vi "Protokoll.vi"() -> ()   [LabVIEW 2015, in "EPA 1065.lvlib" / "Interference verificaton 1065-366.lvlib"]
uses:
  Interference verificaton 1065-366.lvlib
  Allgemein/allgemeine Sub-VIs.lvlib
  Aktion FGV Test.ctl
  Aktion FGV Protokoll.ctl
  <vilib>/Waveform/WDTFileIO.llb/Read Waveform from File.vi
  Visualisierungs Elemente/String - Ausgabefeld.ctl
  Visualisierungs Elemente/Zahlen-Ausgabefeld.ctl
  Visualisierungs Elemente/Button.ctl
panel:
  out "Graph2 2":waveform(dbl)[](graph) caption="Graph2"
  out "Flow-weighted mean":T1
  out "Measured Concentration 3":T1
  out "Measured Concentration 2":T1
  out "Komponente 4":T1 caption="Interferent 3"
  out "Komponente 3":T1 caption="Interferent 2"
  out "Komponente 2":T1 caption="Interferent 1"
  out "Measured Interference %":T1
  in  "Screenshot":T2
  in  "OK":T2
  out "Allowed Interference":T1
  out "Measured Interference":T1
  out "Measured Concentration 1":T1
  out "Target Concentration 3":T1
  out "Target Concentration 2":T1
  out "Target Concentration 1":T1
  out "Datum / Uhrzeit":T1 caption="Date/Time"
  out "Boolesch":bool
  out "Ist Interference":T3 format="%#_5g"
  out "Soll Interference":T3 format="%#_5g"
  out "Konzentration berechnet":T3 caption="Concentration Calculated" format="%#_5g"
  out "Wasserkonzentration":T3 caption="Water-Concentration" format="%#_5g"
  out "Konzentration Feucht":T3 format="%#_5g"
  out "Konzentration Trocken":T3 format="%#_5g"
  out "Komponente":T1 caption="Component"
  out "Bearbeiter":T1 caption="Analyst"
  out "Graph2":waveform(dbl)[](graph)
  # "Interference Test"
  # "Interference Test"
  # "EPA §1065.366\n\nInterference verification of CH4, C2H6,"
  # "Evaluation"
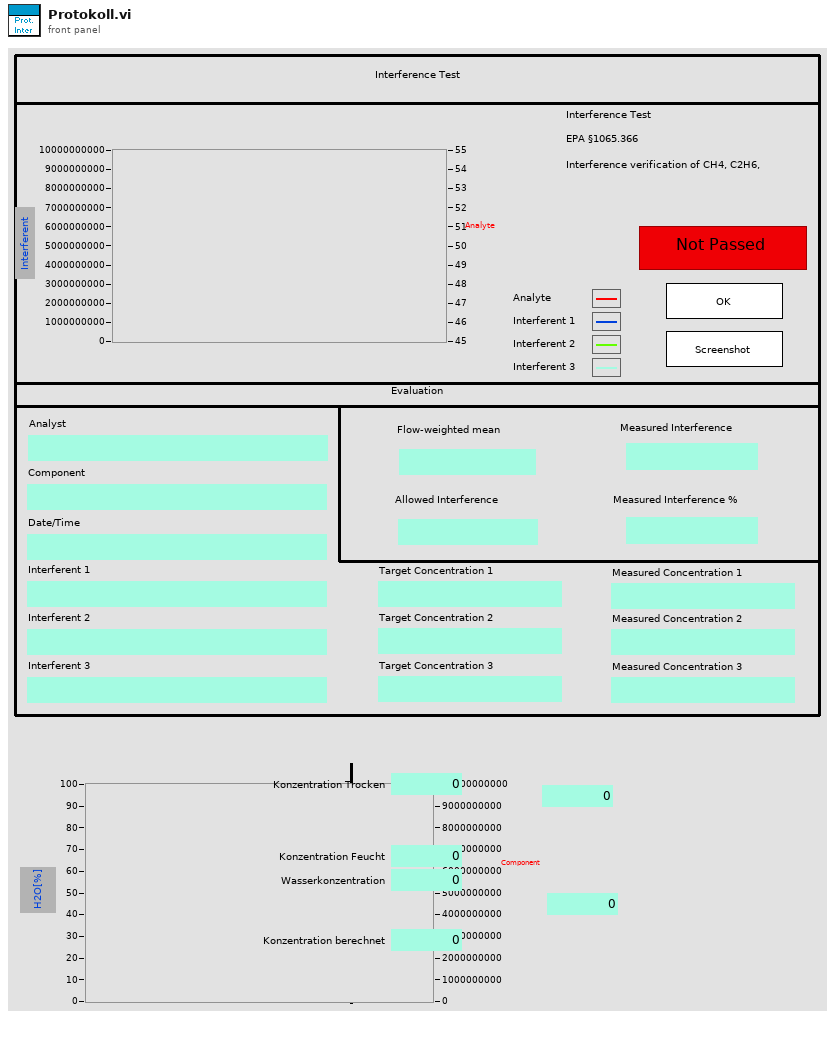
[diagram p1: front panel]
types:
  T1 = typedef "String - Ausgabefeld.ctl" = string
  T2 = typedef "Button.ctl" = bool
  T3 = typedef "Zahlen-Ausgabefeld.ctl" = sgl
  T4 = typedef "EPA 1065.lvlib/Interference verificaton 1065-366.lvlib/Aktion FGV Protokoll.ctl" = enum16{"Lesen", "ini"}
  T5 = typedef "EPA 1065.lvlib/Interference verificaton 1065-366.lvlib/Aktion FGV Test.ctl" = enum16{"Lesen", "ini", "Wasserkonzentration", "Wet", "Dry", "Ergebnis", "Graph", "Interference Daten", "Speichern"}
  T6 = typedef "imagedata.ctl" = cluster{"image type":i32, "image depth":i32, "image":u8[], "mask":u8[], "colors":u32[], "Rectangle":cluster{"left":i16, "top":i16, "right":i16, "bottom":i16}}
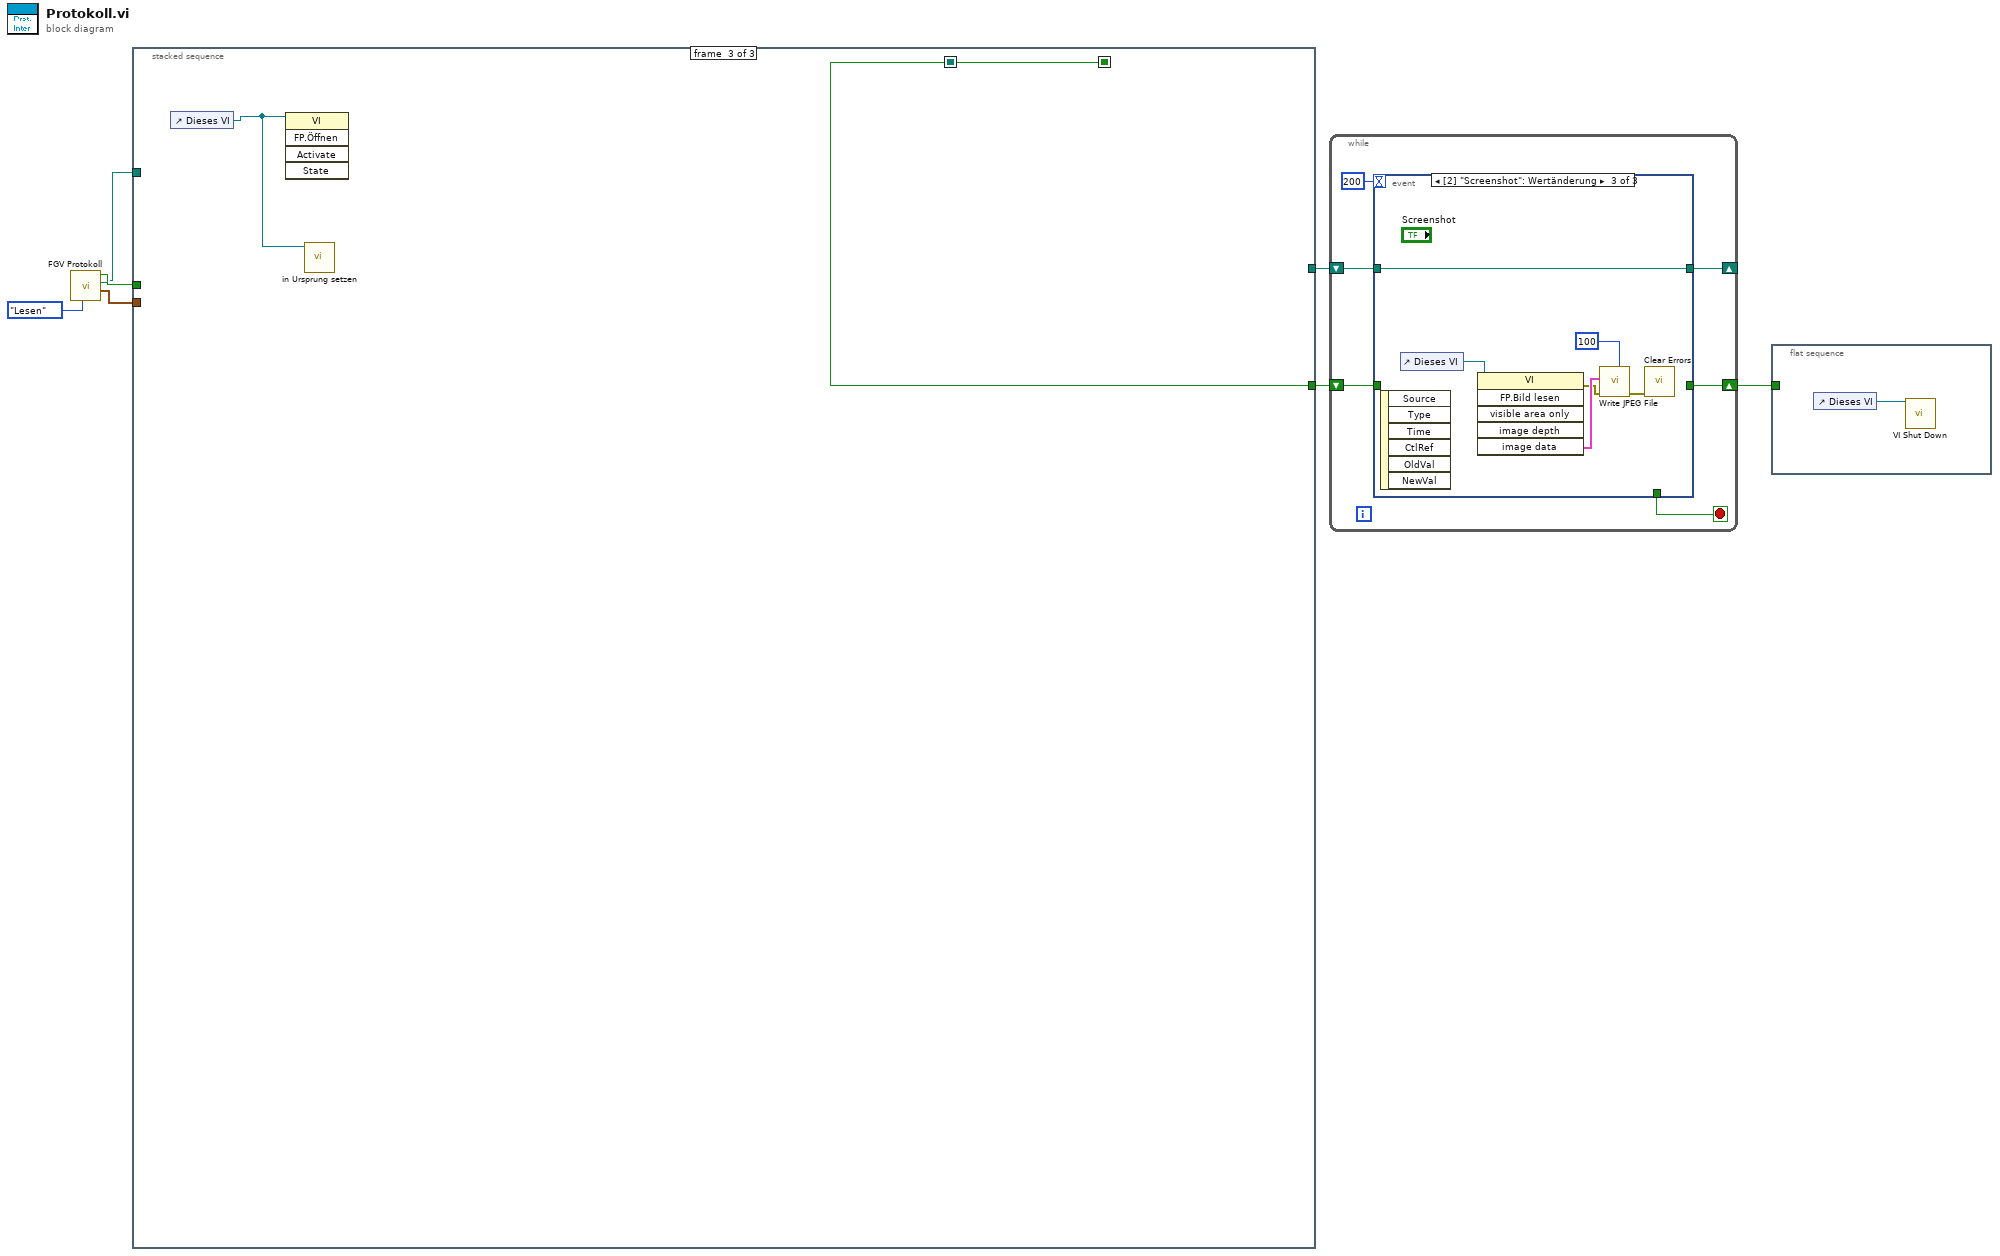
[diagram p0: block diagram]
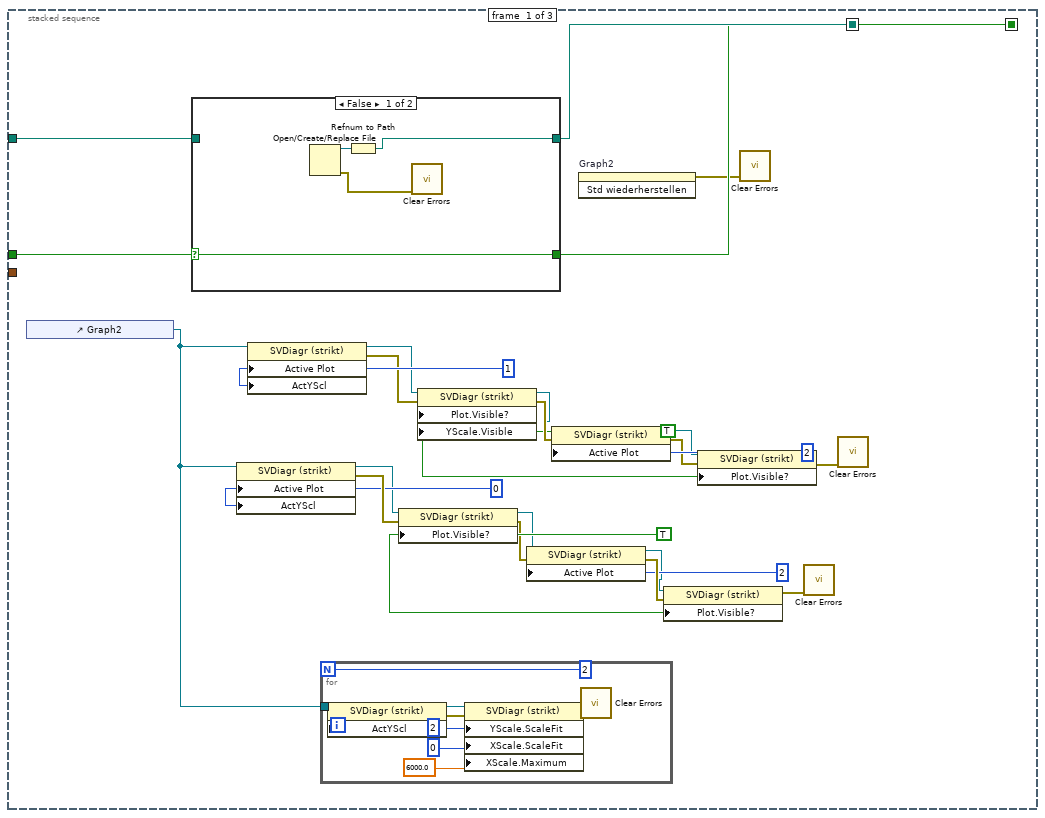
[diagram p2: hidden frame]
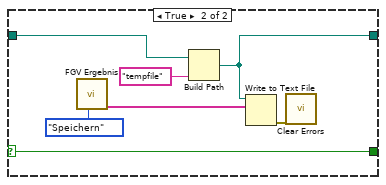
[diagram p3: hidden frame]
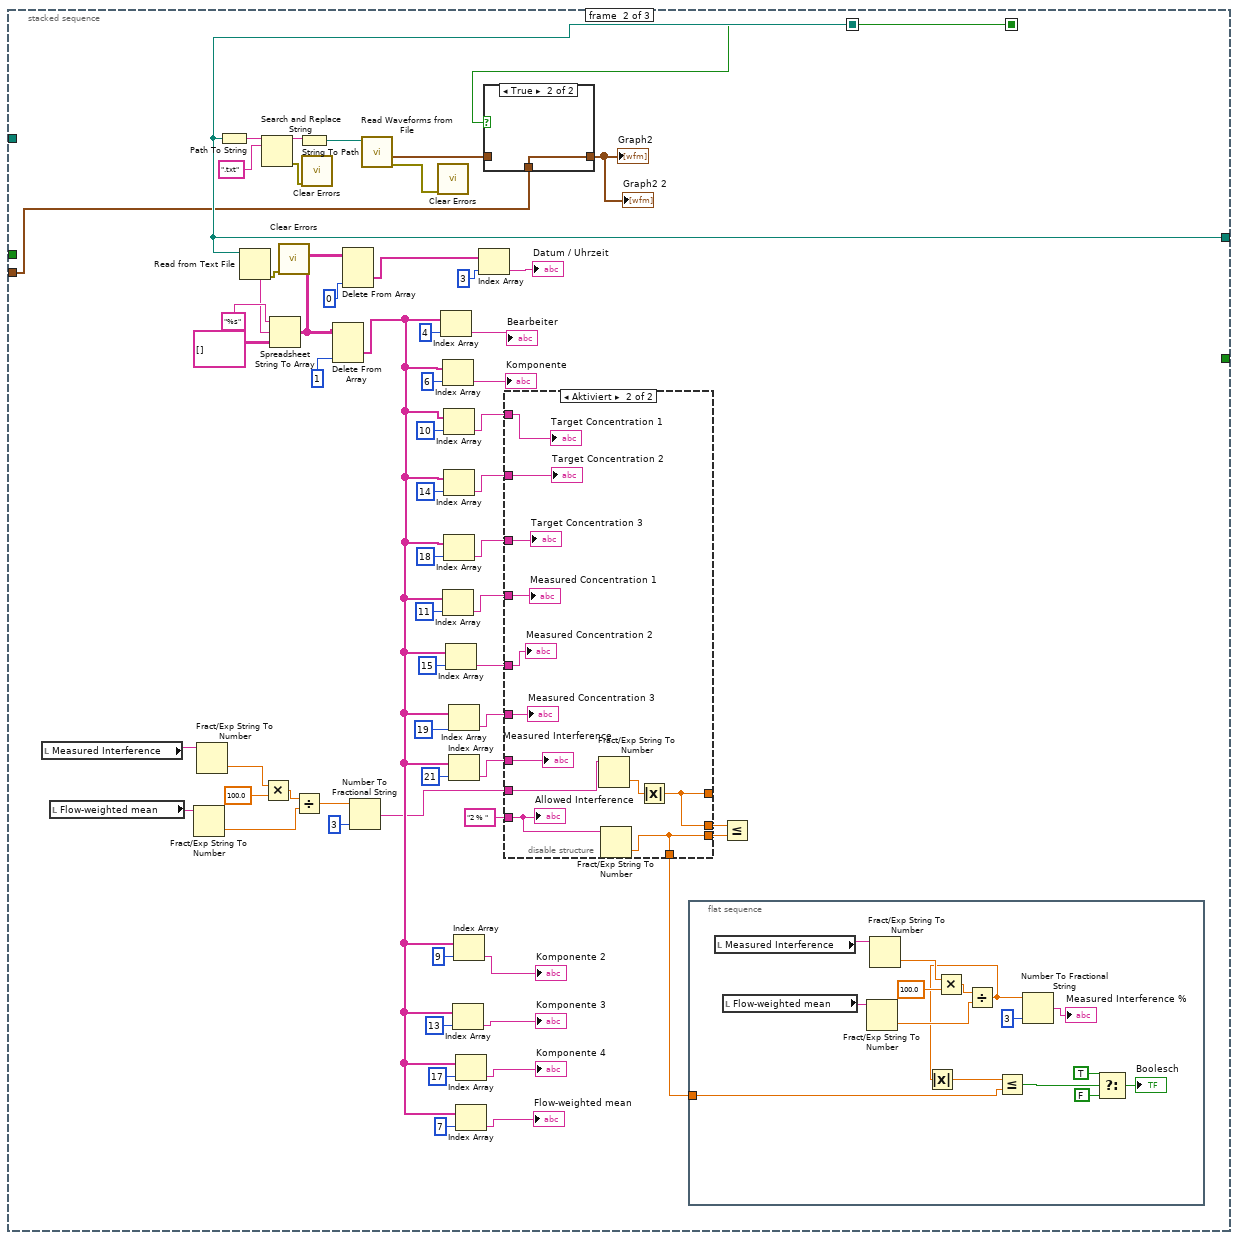
[diagram p4: hidden frame]
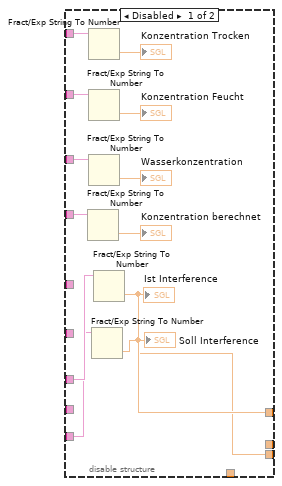
[diagram p6: hidden frame]
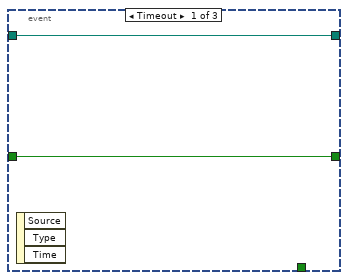
[diagram p7: hidden frame]
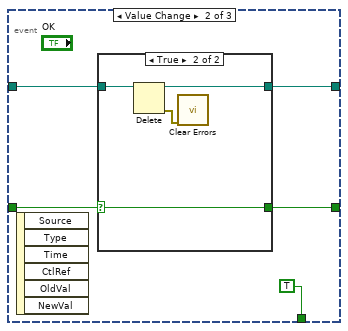
[diagram p8: hidden frame]
diagram:
  n1 = call "FGV Protokoll.vi"("Enum"=Aktion_FGV_Protokoll."Lesen") -> ("Graph2 2"=w1:waveform(dbl)[], "Pfad"=w2:path, "Boolesch 2"=w3:bool)  [unwired: 7 in, 1 out]
  n2 = stacked-sequence {
    seq-local: [w34 _ _] -> [_ w86 _]
    seq-local: [w33 _ _] -> [_ w82 w156]
    tunnel: [_ _ w156] -> w6
    tunnel: [_ w86 _] -> w5
    tunnel: w3 -> [w9 _ _]
    tunnel: w2 -> [w8 _ _]
    tunnel: w1 -> [_ w80 _]
    frame #0 {
      w25 = TRUE ("Plot.Sichtbar")
      w20 = u32 0 ("Aktiver Plot")
      w19 = TRUE ("Plot.Sichtbar")
      w32 = u32 1 ("Aktiver Plot")
      n3 = control-ref of="Graph2"() -> (w18:refnum<vi>)
      n4 = case shown="False" w9 {
        selector: w9 -> [w46 w51]
        tunnel: [w43 w48] -> w34
        tunnel: [w46 w51] -> w33
        tunnel: w8 -> [_ w47]
        frame False {
          n5 = Open/Create/Replace File() -> (refnum out=w45:refnum<file>, error out=w44:errorcluster)  [unwired: 6 in, 1 out]
          n6 = Refnum to Path(1:w45) -> (0:w43:path)
          n7 = call <vilib>:"Clear Errors.vi"("error in (no error)"=w44) -> ()  [unwired: 5 in, 2 out]
        }
        frame True {
          n8 = call "FGV Ergebnis.vi"("Enum"=Aktion_FGV_Test."Speichern") -> ("Protokoll"=w53:T1[])  [unwired: 5 in, 5 out]
          n9 = Build Path(base path=w47, name or relative path="tempfile" ("Name oder relativer Pfad")) -> (appended path=w48:path)
          n10 = Write to Text File(file (use dialog)=w48, text=w53) -> (error out=w50:errorcluster)  [unwired: 2 in, 2 out]
          n11 = call <vilib>:"Clear Errors.vi"("error in (no error)"=w50) -> ()  [unwired: 5 in, 2 out]
        }
      }
      n12 = property on="Eigenschaftsknoten" class="SVDiagr (strikt)"(reference=w18, "Active Plot"=w20, "ActYScl"=w20) -> (reference out=w17:refnum<vi>, error out=w21:errorcluster)  [unwired: 1 in]
      n13 = property on="Eigenschaftsknoten" class="SVDiagr (strikt)"(reference=w18, "Active Plot"=w32, "ActYScl"=w32) -> (reference out=w14:refnum<vi>, error out=w31:errorcluster)  [unwired: 1 in]
      n14 = for {
        N: 2 -> [_]
        tunnel: w18 -> [w36]
        i -> [w42]
        n15 = property on="Eigenschaftsknoten" class="SVDiagr (strikt)"(reference=w36, "ActYScl"=w42) -> (reference out=w35:refnum<vi>, error out=w41:errorcluster)  [unwired: 1 in]
        n16 = property on="Eigenschaftsknoten" class="SVDiagr (strikt)"(reference=w35, error in=w41, "YScale.ScaleFit"=u8 2 ("Y-Achse.Achsenanpassung"), "XScale.ScaleFit"=u8 0 ("X-Achse.Achsenanpassung"), "XScale.Maximum"=6000.0 ("X-Achse.Bereich:Maximum")) -> (error out=w40:errorcluster)  [unwired: 1 out]
        n17 = call <vilib>:"Clear Errors.vi"("error in (no error)"=w40) -> ()  [unwired: 5 in, 2 out]
      }
      n18 = property on="Eigenschaftsknoten" class="SVDiagr (strikt)"(reference=w17, error in=w21, "Plot.Visible?"=w25) -> (reference out=w16:refnum<vi>, error out=w22:errorcluster)
      n19 = property on="Eigenschaftsknoten" class="SVDiagr (strikt)"(reference=w14, error in=w31, "Plot.Visible?"=w19, "YScale.Visible"=w19) -> (reference out=w13:refnum<vi>, error out=w30:errorcluster)
      n20 = property on="Eigenschaftsknoten" class="SVDiagr (strikt)"(reference=w16, error in=w22, "Active Plot"=u32 2 ("Aktiver Plot")) -> (reference out=w15:refnum<vi>, error out=w24:errorcluster)
      n21 = property on="Eigenschaftsknoten" class="SVDiagr (strikt)"(reference=w13, error in=w30, "Active Plot"=u32 2 ("Aktiver Plot")) -> (reference out=w12:refnum<vi>, error out=w28:errorcluster)
      n22 = invoke on="Graph2" class="SVDiagr (strikt)" method="Std wiederherstellen"() -> (error out=w10:errorcluster)  [unwired: 3 in, 2 out]
      n23 = property on="Eigenschaftsknoten" class="SVDiagr (strikt)"(reference=w15, error in=w24, "Plot.Visible?"=w25) -> (error out=w26:errorcluster)  [unwired: 1 out]
      n24 = property on="Eigenschaftsknoten" class="SVDiagr (strikt)"(reference=w12, error in=w28, "Plot.Visible?"=w19) -> (error out=w27:errorcluster)  [unwired: 1 out]
      n25 = call <vilib>:"Clear Errors.vi"("error in (no error)"=w10) -> ()  [unwired: 5 in, 2 out]
      n26 = call <vilib>:"Clear Errors.vi"("error in (no error)"=w26) -> ()  [unwired: 5 in, 2 out]
      n27 = call <vilib>:"Clear Errors.vi"("error in (no error)"=w27) -> ()  [unwired: 5 in, 2 out]
    }
    frame #1 {
      n28 = local read "Measured Interference"() -> (w64:T1)
      n29 = local read "Flow-weighted mean"() -> (w65:T1)
      n30 = Fract/Exp String To Number(string=w65) -> (number=w60:dbl)  [unwired: 3 in, 1 out]
      n31 = Fract/Exp String To Number(string=w64) -> (number=w61:dbl)  [unwired: 3 in, 1 out]
      n32 = Path To String(path=w86) -> (string=w90:string)
      n33 = Read from Text File(file (use dialog)=w86) -> (text=w92:string, error out=w114:errorcluster)  [unwired: 2 in, 3 out]
      n34 = Search and Replace String(input string=w90, search string=".txt" ("Such-String")) -> (result string=w88:string, error out=w54:errorcluster)  [unwired: 6 in, 2 out]
      n35 = Multiply(x=w61, y=sgl 100.0) -> (x*y=w62:dbl)
      n36 = Spreadsheet String To Array(format string="%s" ("Format-String"), spreadsheet string=w92, array type (2D Dbl)=string[][] []) -> (array=w81:string[][])  [unwired: 1 out]
      n37 = call <vilib>:"Clear Errors.vi"("error in (no error)"=w114) -> ()  [unwired: 5 in, 2 out]
      n38 = Divide(x=w62, y=w60) -> (x/y=w59:dbl)
      n39 = String To Path(string=w88) -> (path=w87:path)
      n40 = call <vilib>:"Clear Errors.vi"("error in (no error)"=w54) -> ()  [unwired: 5 in, 2 out]
      n41 = Delete From Array(array=w81, index (col)=1 ("Deaktivierter Index (Zeile)")) -> (deleted portion=w66:string[])  [unwired: 2 in, 1 out]
      n42 = Delete From Array(array=w81, index (col)=0 ("Deaktivierter Index (Spalte)")) -> (deleted portion=w95:string[])  [unwired: 2 in, 1 out]
      n43 = Number To Fractional String(number=w59, precision (6)=i16 3 ("Genauigkeit (6)")) -> (F-format string=w56:string)  [unwired: 2 in]
      n44 = call-poly <vilib>:"Read Waveforms from File.vi"("file path (dialog if empty)"=w87) -> ("error out"=w85:errorcluster, "all waveforms in record"=w83:waveform(dbl)[])  [unwired: 5 in, 2 out]
      n45 = call <vilib>:"Clear Errors.vi"("error in (no error)"=w85) -> ()  [unwired: 5 in, 2 out]
      n46 = Index Array(array=w66, index=4 ("Index (Zeile)")) -> (element=→"Bearbeiter":string)
      n47 = Index Array(array=w66, index=6 ("Index")) -> (element=→"Komponente":string)
      n48 = Index Array(array=w66, index=11 ("Index")) -> (element=w109:string)
      n49 = Index Array(array=w66, index=10 ("Index")) -> (element=w104:string)
      n50 = Index Array(array=w66, index=14 ("Index")) -> (element=w105:string)
      n51 = Index Array(array=w66, index=18 ("Index")) -> (element=w108:string)
      n52 = Index Array(array=w66, index=15 ("Index")) -> (element=w72:string)
      n53 = Index Array(array=w66, index=19 ("Index")) -> (element=w70:string)
      n54 = Index Array(array=w66, index=21 ("Index")) -> (element=w112:string)
      n55 = Index Array(array=w66, index=13 ("Index")) -> (element=→"Komponente 3":string)
      n56 = Index Array(array=w66, index=9 ("Index")) -> (element=→"Komponente 2":string)
      n57 = Index Array(array=w66, index=17 ("Index")) -> (element=→"Komponente 4":string)
      n58 = Index Array(array=w66, index=7 ("Index")) -> (element=→"Flow-weighted mean":string)
      n59 = Index Array(array=w95, index=3 ("Deaktivierter Index (Spalte)")) -> (element=→"Datum / Uhrzeit":string)
      n60 = case shown="True" w82 {
        tunnel: [w130 w131] -> w57
        tunnel: w83 -> [w130 _]
        tunnel: w80 -> [_ w131]
        frame False {
        }
        frame True {
        }
      }
      "Graph2" <- w57
      "Graph2 2" <- w57
      n61 = disable-structure shown="Aktiviert" {
        disable-tunnel: w104 -> [w142 w155]
        disable-tunnel: w105 -> [w141 w154]
        disable-tunnel: w108 -> [w139 w153]
        disable-tunnel: w109 -> [w137 w152]
        disable-tunnel: w112 -> [w135 w151]
        disable-tunnel: "2 % " -> [w134 w150]
        disable-tunnel: [w133 w148] -> _
        disable-tunnel: [w132 w144] -> w113
        disable-tunnel: [_ w148] -> w84
        disable-tunnel: w72 -> [_ w147]
        disable-tunnel: w70 -> [_ w146]
        disable-tunnel: w56 -> [_ w145]
        disable-tunnel: [_ w144] -> w55
        frame Disabled {
          n62 = Fract/Exp String To Number(string=w137) -> (number=→"Konzentration berechnet":dbl)  [unwired: 3 in, 1 out]
          n63 = Fract/Exp String To Number(string=w142) -> (number=→"Konzentration Trocken":dbl)  [unwired: 3 in, 1 out]
          n64 = Fract/Exp String To Number(string=w141) -> (number=→"Konzentration Feucht":dbl)  [unwired: 3 in, 1 out]
          n65 = Fract/Exp String To Number(string=w139) -> (number=→"Wasserkonzentration":dbl)  [unwired: 3 in, 1 out]
          n66 = Fract/Exp String To Number(string=w134) -> (number=w132:dbl)  [unwired: 3 in, 1 out]
          "Soll Interference" <- w132
          n67 = Fract/Exp String To Number(string=w135) -> (number=w133:dbl)  [unwired: 3 in, 1 out]
          "Ist Interference" <- w133
        }
        frame Enabled {
          n68 = Fract/Exp String To Number(string=w145) -> (number=w149:dbl)  [unwired: 3 in, 1 out]
          n69 = Fract/Exp String To Number(string=w150) -> (number=w144:dbl)  [unwired: 3 in, 1 out]
          n70 = Absolute Value(x=w149) -> (abs(x)=w148:dbl)
          "Allowed Interference" <- w150
          "Measured Interference" <- w151
          "Target Concentration 1" <- w155
          "Target Concentration 2" <- w154
          "Target Concentration 3" <- w153
          "Measured Concentration 1" <- w152
          "Measured Concentration 2" <- w147
          "Measured Concentration 3" <- w146
        }
      }
      n71 = flat-sequence {
        tunnel: w55 -> [w119]
        frame #0 {
          n72 = local read "Measured Interference"() -> (w124:T1)
          n73 = local read "Flow-weighted mean"() -> (w123:T1)
          n74 = Fract/Exp String To Number(string=w123) -> (number=w128:dbl)  [unwired: 3 in, 1 out]
          n75 = Fract/Exp String To Number(string=w124) -> (number=w127:dbl)  [unwired: 3 in, 1 out]
          n76 = Multiply(x=w127, y=sgl 100.0) -> (x*y=w126:dbl)
          n77 = Divide(x=w126, y=w128) -> (x/y=w121:dbl)
          n78 = Absolute Value(x=w121) -> (abs(x)=w120:dbl)
          n79 = Less Or Equal?(x=w120, y=w119) -> (x <= y?=w115:bool)
          n80 = Number To Fractional String(number=w121, precision (6)=i16 3 ("Genauigkeit (6)")) -> (F-format string=→"Measured Interference %":string)  [unwired: 2 in]
          n81 = Select(t=TRUE, s=w115, f=FALSE) -> (s? t:f=→"Boolesch":bool)
        }
      }
      n82 = Less Or Equal?(x=w84, y=w113) -> ()  [unwired: 1 out]
    }
    frame #2 {
      n83 = control-ref of="Dieses VI"() -> (w157:refnum<vi>)
      n84 = invoke class="VI" method="FP.Öffnen"(reference=w157) -> ()  [unwired: 4 in, 5 out]
      n85 = call "in Ursprung setzen.vi"("VI Referenz"=w157) -> ()  [unwired: 11 in]
    }
  }
  n86 = while {
    shift-right: [w163] -> _
    shift-left: w5 -> [w162]
    shift-right: [w161] -> w7
    shift-left: w6 -> [w160]
    stop <- w158 stop-if-true
    n87 = event shown="[2] \"Screenshot\": Wertänderung" {
      selector: _ -> [_ _ _]
      dyn-events: _ -> [_ _ _]
      timeout: 200 -> [_ _ _]
      tunnel: [w165 w167 w178] -> w163
      tunnel: w162 -> [w165 w170 w178]
      tunnel: w160 -> [w164 w169 _]
      tunnel: [w164 w168 _] -> w161
      tunnel: [_ TRUE _] -> w158
      event Timeout {
        n88 = event-data() -> ()  [unwired: 1 in, 3 out]
      }
      event Value Change {
        n89 = event-data() -> ()  [unwired: 1 in, 6 out]
        n90 = case shown="True" w169 {
          selector: w169 -> [w172 w175]
          tunnel: w170 -> [w171 w176]
          tunnel: [w172 w175] -> w168
          tunnel: [w171 w174] -> w167
          frame False {
          }
          frame True {
            n91 = Delete(path (use dialog)=w176) -> (deleted path=w174:path, error out=w173:errorcluster)  [unwired: 4 in, 1 out]
            n92 = call <vilib>:"Clear Errors.vi"("error in (no error)"=w173) -> ()  [unwired: 5 in, 2 out]
          }
        }
      }
      event Value Change {
        n93 = event-data() -> ()  [unwired: 1 in, 6 out]
        n94 = control-ref of="Dieses VI"() -> (w182:refnum<vi>)
        n95 = invoke class="VI" method="FP.Bild lesen"(reference=w182) -> (error out=w180:errorcluster, "image data"=w181:T6)  [unwired: 5 in, 4 out]
        n96 = call <vilib>:"Write JPEG File.vi"("quality (80)"=100, "error in (no error)"=w180, "image data"=w181) -> ("error out"=w179:errorcluster)  [unwired: 7 in, 1 out]
        n97 = call <vilib>:"Clear Errors.vi"("error in (no error)"=w179) -> ()  [unwired: 5 in, 2 out]
      }
    }
  }
  n98 = flat-sequence {
    tunnel: w7 -> [_]
    frame #0 {
      n99 = control-ref of="Dieses VI"() -> (w183:refnum<vi>)
      n100 = call "VI Shut Down.vi"("VI Referenz"=w183) -> ()  [unwired: 11 in]
    }
  }
